vi "Node - Configure.vi"(8 "error in (no error)":errorcluster, 10 "Node Configuration Properties In":T1) -> (0 "error out":errorcluster, 2 "Node Configuration Properties Out":T1, 3 "Node Data":T3)   [LabVIEW 2016, in "PXImc Router.lvlib"]
uses:
  PXImc Router.lvlib
  Controls/Node - Configuration.ctl
  Controls/Table Index-Size.ctl
  Controls/Node Data.ctl
  <vilib>/pximc/Initialize Reader Session (DBL).vi
  <vilib>/pximc/Initialize Writer Session (DBL).vi
  <vilib>/pximc/nipximc.lvlib
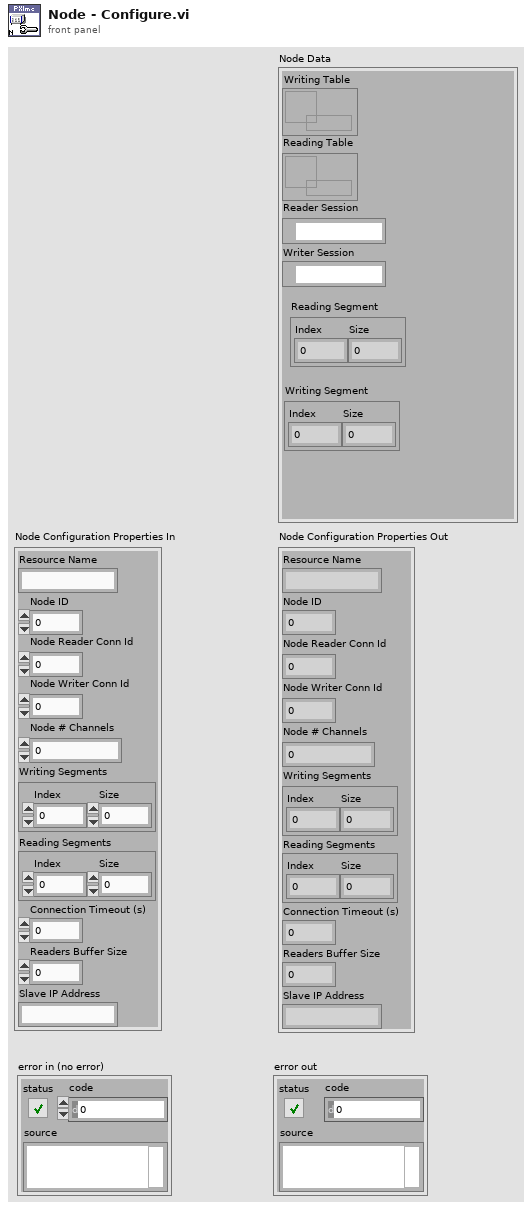
[diagram p1: front panel]
types:
  T1 = typedef "PXImc Router.lvlib/Node - Configuration.ctl" = cluster{"Resource Name":string, "Node ID":u16, "Node Reader Conn Id":u16, "Node Writer Conn Id":u16, "Node # Channels":u32, "Writing Segments":T2, "Reading Segments":T2, "Connection Timeout (s)":dbl, "Readers Buffer Size":u32, "Slave IP Address":string}
  T2 = typedef "PXImc Router.lvlib/Table Index-Size.ctl" = cluster{"Index":u32, "Size":u32}
  T3 = typedef "PXImc Router.lvlib/Node Data.ctl" = cluster{"Writing Table":refnum<data-value>, "Reading Table":refnum<data-value>, "Reader Session":refnum<k21>, "Writer Session":refnum<k21>, "Reading Segment":T2, "Writing Segment":T2}
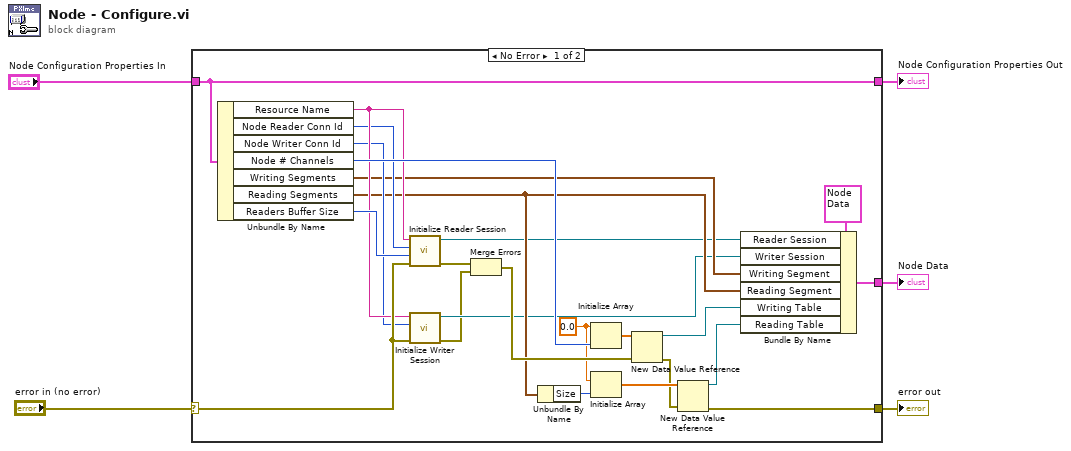
[diagram p0: block diagram]
diagram:
  n1 = case shown="No Error" "error in (no error)" {
    selector: "error in (no error)" -> [w26 w31]
    tunnel: [w29 _] -> w2
    tunnel: [w15 w31] -> w5
    tunnel: "Node Configuration Properties In" -> [w6 w30]
    tunnel: [w6 w30] -> w1
    frame No Error {
      w13 = 0.0 ("element")
      n2 = Unbundle By Name(w6) -> ("Resource Name"=w23:string, "Node Reader Conn Id"=w22:u16, "Node Writer Conn Id"=w21:u16, "Node # Channels"=w24:u32, "Writing Segments"=w19:T2, "Reading Segments"=w12:T2, "Readers Buffer Size"=w25:u32)
      n3 = call-poly <vilib>:"Initialize Reader Session.vi"("error in (no error)"=w26, "buffer size"=w25, "writer's connection id (1)"=w22, "interface"=w23) -> ("error out"=w7:errorcluster, "session out"=w10:refnum<k21>)  [unwired: 6 in]
      n4 = call-poly <vilib>:"Initialize Writer Session.vi"("error in (no error)"=w26, "connection id (1)"=w21, "interface"=w23) -> ("error out"=w8:errorcluster, "session out"=w9:refnum<k21>)  [unwired: 7 in]
      n5 = Merge Errors(w7, w8) -> (w18:errorcluster)
      n6 = Unbundle By Name(w12) -> ("Size"=w11:u32)
      n7 = Initialize Array(w13, w24) -> (w27:dbl[])
      n8 = Initialize Array(w13, w11) -> (w17:dbl[])
      n9 = New Data Value Reference(data value=w27, error in=w18) -> (data value reference=w28:refnum<data-value>, error out=w16:errorcluster)
      n10 = New Data Value Reference(data value=w17, error in=w16) -> (data value reference=w14:refnum<data-value>, error out=w15:errorcluster)
      n11 = Bundle By Name(cluster=T3 {"Writing Table"=refnum, "Reading Table"=refnum, "Reader Session"="", "Writer Session"="", "Reading Segment"={"Index"=0, "Size"=0}, "Writing Segment"={"Index"=0, "Size"=0}} ("Router Data"), "Reader Session"=w10, "Writer Session"=w9, "Writing Segment"=w19, "Reading Segment"=w12, "Writing Table"=w28, "Reading Table"=w14) -> (w29:T3)
    }
    frame Error {
    }
  }
  "error out" <- w5
  "Node Data" <- w2
  "Node Configuration Properties Out" <- w1
